vi "CheesyDrive.vi"(6 "Quickturn":bool, 7 "SlowMode":bool, 10 "Wheel":dbl(slide) scale=-1.0..1.0, 11 "Throttle":dbl(slide)=0.007874015748031496 scale=-1.0..1.0) -> (2 "Right PWM":dbl, 3 "Left PWM":dbl)   [LabVIEW 2017]
doc: "Implements CheesyDrive. CheesyDrive means that the turn joystick controls the radius of turning instead of the rate of turning. Also implements QuickStop and QuickTurn."
panel:
  in  "MaxSpeedTurnNotQuick":dbl=10.0 format="%#_13g"
  in  "MaxTurnRateSlow":dbl=20.0
  in  "MaxTurnSlow":dbl=0.55
  in  "MaxSpeedSlow":dbl=0.5
  in  "SlowRate":dbl=1.0
  in  "PointsTurn":cluster{"X":dbl, "Y":dbl}[](array[cluster])=[{"X"=0.0, "Y"=0.0}, {"X"=0.04, "Y"=0.0}, {"X"=0.041, "Y"=0.01}, {"X"=1.0, "Y"=1.0}]
  in  "PointsQuickTurn":cluster{"X":dbl, "Y":dbl}[](array[cluster])=[{"X"=0.0, "Y"=0.0}, {"X"=0.04, "Y"=0.0}, {"X"=0.041, "Y"=0.2}, {"X"=0.5, "Y"=0.5}, {"X"=1.0, "Y"=1.0}]
  in  "PointsThrottle":cluster{"X":dbl, "Y":dbl}[](array[cluster])=[{"X"=0.0, "Y"=0.0}, {"X"=0.04, "Y"=0.0}, {"X"=0.0251, "Y"=0.15}, {"X"=1.0, "Y"=1.0}]
  in  "CarLikeTurning":bool
  in  "QSMult":dbl=0.1
  in  "WheelNonLinearity":dbl=0.65
  in  "negInertiaScalar":dbl=3.0
  in  "MaxRate":dbl=7.0
  in  "alpha":dbl=0.1
  out "Waveform Chart":dbl(graph)
  in  "Sensitivty":dbl=1.0
  # "Enable to enable"
  # "(for quickstop decay)"
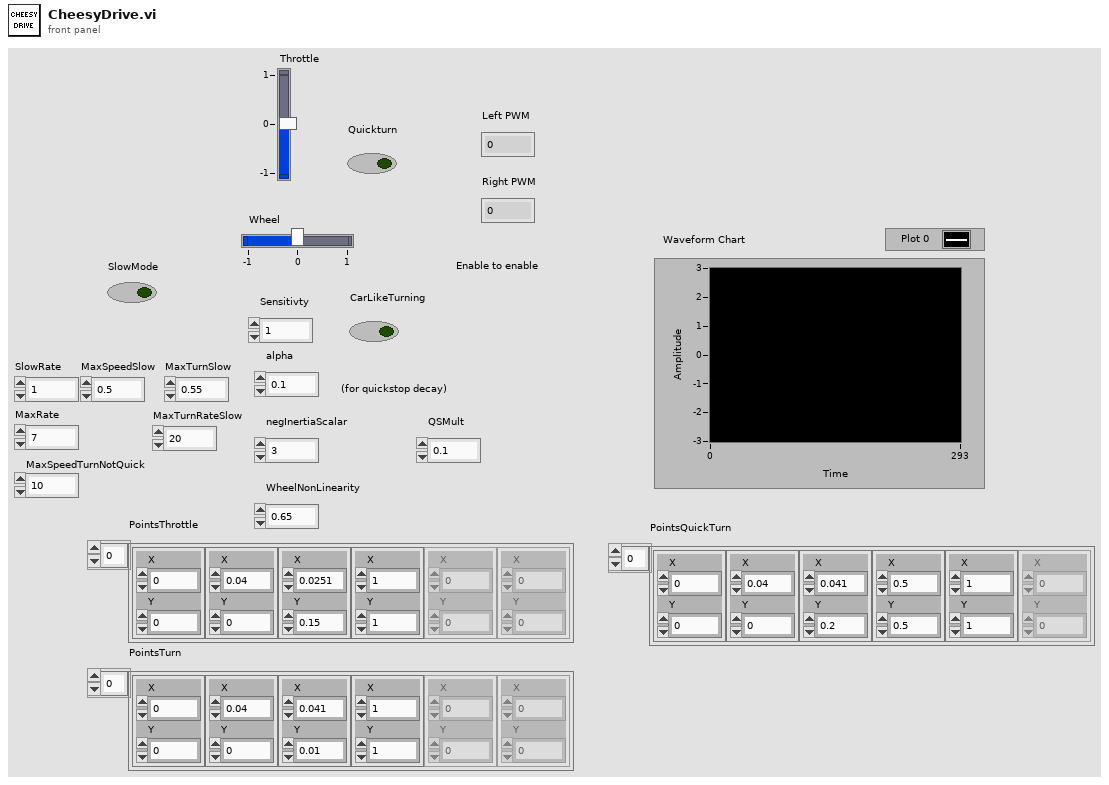
[diagram p1: front panel]
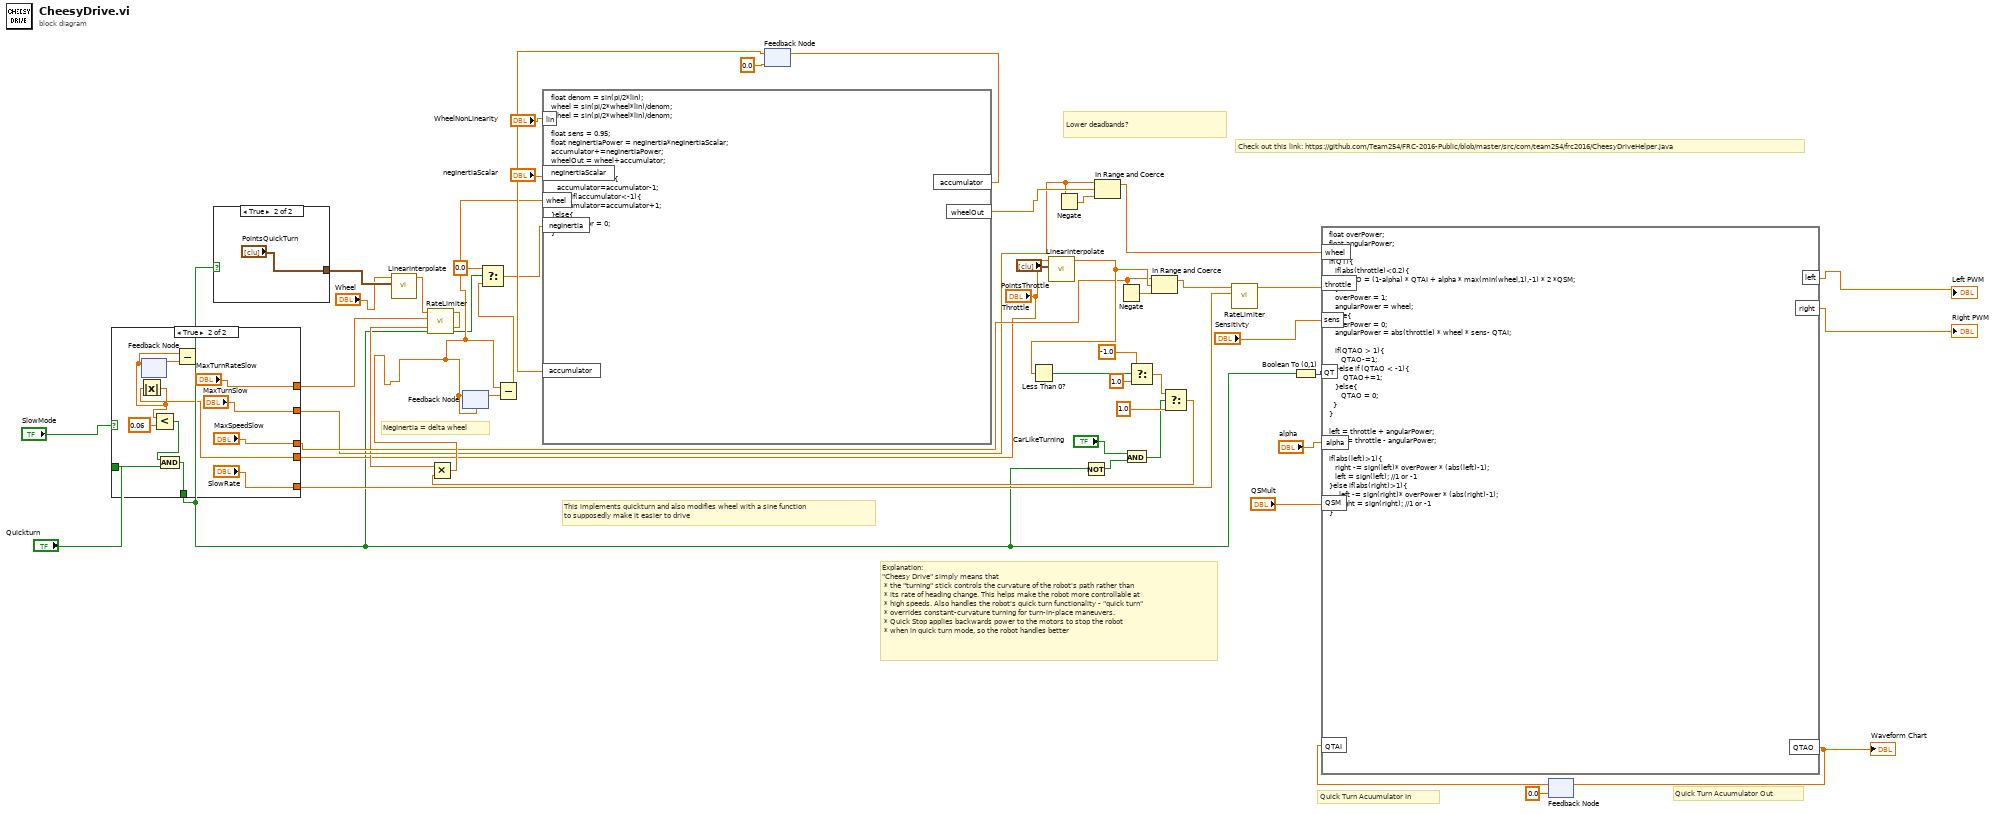
[diagram p0: block diagram]
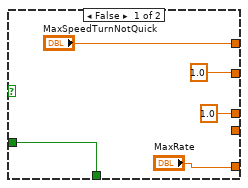
[diagram p2: hidden frame]
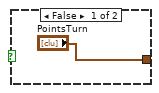
[diagram p3: hidden frame]
diagram:
  # "This implements quickturn and also modifies wheel with a sine function\nto supposedly make it easier to drive"
  # "Lower deadbands?"
  # "NegInertia = delta wheel"
  # "Explanation:\n\"Cheesy Drive\" simply means that\n * the \"turning\" stick controls the curvature of the robot's path rather than\n * its rate of heading change. This helps make the robot more controllable at\n * high speeds. Also handles the robot's quick turn functionality - \"quick turn\"\n * overrides constant-curvature turning for turn-in-place maneuvers.\n * Quick Stop applies backwards power to the motors to stop the robot\n * when in quick turn mode, so the robot handles better"
  # "Quick Turn Acuumulator Out"
  # "Quick Turn Acuumulator In"
  # "Check out this link: https://github.com/Team254/FRC-2016-Public/blob/master/src/com/team254/frc2016/CheesyDriveHelper.java"
  n1 = case shown="True" "SlowMode" {
    tunnel: ["MaxRate" "SlowRate"] -> w20
    tunnel: [1.0 ("MaxSpeedSlow") "MaxSpeedSlow"] -> w17
    tunnel: [1.0 ("MaxSpeedSlow") "MaxTurnSlow"] -> w14
    tunnel: ["MaxSpeedTurnNotQuick" "MaxTurnRateSlow"] -> w11
    tunnel: "Quickturn" -> [w49 w60]
    tunnel: [w49 w57] -> w1
    tunnel: "Throttle" -> [_ w56]
    frame False {
    }
    frame True {
      n2 = Absolute Value(x=w56) -> (abs(x)=w54:dbl)
      n3 = feedback-in #1(w54) -> ()
      n4 = feedback #1() -> (w55:dbl)  [unwired: 1 in]
      n5 = Less?(x=w54, y=0.06) -> (x < y?=w59:bool)
      n6 = And(x=w59, y=w60) -> (x .and. y?=w57:bool)
      n7 = Subtract(x=w54, y=w55) -> ()  [unwired: 1 out]
    }
  }
  n8 = case shown="True" w1 {
    tunnel: ["PointsTurn" "PointsQuickTurn"] -> w22
    frame False {
    }
    frame True {
    }
  }
  n9 = call "LinearInterpolate.vi"("Points"=w22, "Value"="Wheel") -> ("Output"=w13:dbl)  [unwired: 9 in]
  n10 = call "RateLimiter.vi"("Max dx/dt"=w11, "Input"=w13) -> ("Output"=w12:dbl)  [unwired: 9 in]
  n11 = feedback #2(0.0 ("Wheel")) -> (w38:dbl)
  n12 = call "LinearInterpolate.vi"("Points"="PointsThrottle", "Value"="Throttle") -> ("Output"=w19:dbl)  [unwired: 9 in]
  n13 = Less Than 0?(x=w19) -> (x < 0?=w30:bool)
  n14 = Negate(x=w14) -> (-x=w15:dbl)
  n15 = Not(x=w1) -> (.not. x?=w3:bool)
  n16 = Negate(x=w17) -> (-x=w18:dbl)
  n17 = And(x="CarLikeTurning", y=w3) -> (x .and. y?=w2:bool)
  n18 = Select(t=-1.0, s=w30, f=1.0) -> (s? t:f=w26:dbl)
  n19 = In Range and Coerce(upper limit=w17, x=w19, lower limit=w18) -> (coerced(x)=w16:dbl)  [unwired: 1 out]
  n20 = Select(t=w26, s=w2, f=1.0) -> (s? t:f=w24:dbl)
  n21 = Multiply(x=w12, y=w24) -> (x*y=w27:dbl)
  n22 = feedback #3(w27) -> (w39:dbl)
  n23 = feedback-in #3(w27) -> ()
  n24 = Subtract(x=w27, y=w39) -> (x-y=w9:dbl)
  n25 = Select(t=0.0, s=w1, f=w9) -> (s? t:f=w10:dbl)
  n26 = formula code="float denom = sin(pi/2*lin);\nwheel = sin(pi/2*wheel*lin)/denom;\nwheel = sin(pi/2*wheel*lin)/denom;\n\nfloat sens = 0.95;\nfloat negInertiaPower = negInertia*negInertiaScalar;\naccumulator+=negInertiaPower;\nwheelOut = wheel+accumulator;\n\nif(accumulator>1){\n   accumulator=accumulator-1;\n}else if(accumulator<-1){\n   accumulator=accumulator+1;\n}else{\naccumulator = 0;\n}"("wheel"=w27, "negInertia"=w10, "accumulator"=w38, "negInertiaScalar"="negInertiaScalar", "lin"="WheelNonLinearity") -> ("accumulator"=w36:dbl, "wheelOut"=w32:dbl)
  n27 = feedback-in #2(w36) -> ()
  n28 = In Range and Coerce(upper limit=w14, x=w32, lower limit=w15) -> (coerced(x)=w33:dbl)  [unwired: 1 out]
  n29 = call "RateLimiter.vi"("Max dx/dt"=w20, "Input"=w16) -> ("Output"=w42:dbl)  [unwired: 9 in]
  n30 = Boolean To (0,1)(Boolean=w1) -> (0, 1=w46:i16)
  n31 = feedback #4(0.0 ("QTAccumulatorO")) -> (w44:dbl)
  n32 = formula code="float overPower;\nfloat angularPower;\n\nif(QT){\n   if(abs(throttle)<0.2){\n      QTAO = (1-alpha) * QTAI + alpha * max(min(wheel,1),-1) * 2 *QSM;\n   }\n   overPower = 1;\n   angularPower = wheel;\n}else{\n   overPower = 0;\n   angularPower = abs(throttle) * wheel * sens- QTAI;\n\n   if(QTAO > 1){\n      QTAO-=1;\n   }else if (QTAO < -1){\n       QTAO+=1;\n   }else{\n      QTAO = 0;\n  }\n}\n\nleft = throttle + angularPower;\nright = throttle - angularPower;\n\nif(abs(left)>1){\n   right -= sign(left)* overPower * (abs(left)-1);\n   left = sign(left); //1 or -1\n}else if(abs(right)>1){\n     left -= sign(right)* overPower * (abs(right)-1);\n     right = sign(right); //1 or -1 \n}"("wheel"=w33, "throttle"=w42, "sens"="Sensitivty", "QT"=w46, "alpha"="alpha", "QTAI"=w44, "QSM"="QSMult") -> ("left"=→"Left PWM":dbl, "right"=→"Right PWM":dbl, "QTAO"=w47:dbl)
  "Waveform Chart" <- w47
  n33 = feedback-in #4(w47) -> ()
